vi "Extract message by Rotator.vi"(8 "error in (no error)":errorcluster, 9 "timeout in ms (-1)":i32=-1, 10 "Initialized?":bool, 11 "Queue in":refnum<queue>) -> (0 "error out":errorcluster, 1 "Unread":i32, 2 "Data":variant, 3 "Command out":T1)   [LabVIEW 2024, in "SampleRotator.lvlib"]
doc: "Opens message send by top/master contoller. Reads command and if module was not initialized, it will change any other command than \"Initialize\" into \"Ignore\". \n\nInputs:\nmailbox ref; Initialized?; timeout; error cluster\n\nOutputs:\nCommand; Data; number of unread messages; error cluster"
uses:
  SampleRotator.lvlib
  ctl/Rotator commands.ctl
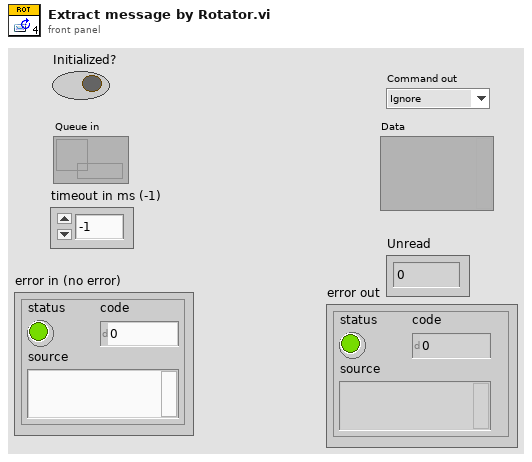
[diagram p1: front panel]
types:
  T1 = typedef "SampleRotator.lvlib/Rotator commands.ctl" = enum16{"Ignore", "Initialize", "Update", "Set parameters", "Stop movement", "Set position", "Disconnect", "End"}
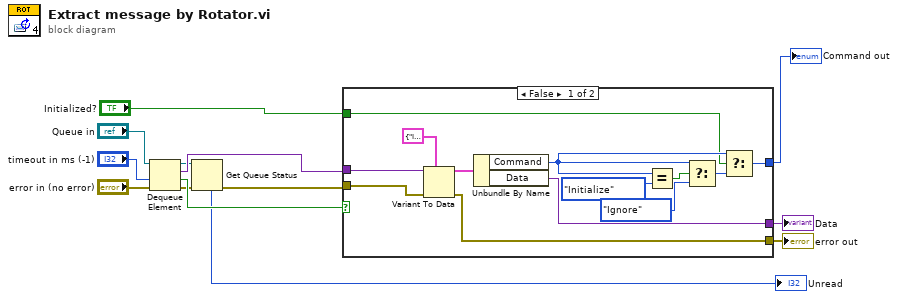
[diagram p0: block diagram]
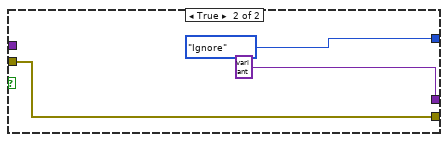
[diagram p2: hidden frame]
diagram:
  n1 = Dequeue Element(queue="Queue in", timeout in ms (-1)="timeout in ms (-1)", error in (no error)="error in (no error)") -> (queue out=w1:refnum<queue>, element=w10:variant, timed out?=w9:bool, error out=w2:errorcluster)
  n2 = Get Queue Status(queue=w1, error in (no error)=w2) -> (error out=w11:errorcluster, # elements in queue=→"Unread":i32)  [unwired: 1 in, 6 out]
  n3 = case shown="False" w9 {
    tunnel: w11 -> [w26 w27]
    tunnel: [w25 w27] -> w3
    tunnel: [w24 variant ("Data")] -> w5
    tunnel: [w23 Rotator_commands."Ignore" ("Command in")] -> w13
    tunnel: w10 -> [w19 _]
    tunnel: "Initialized?" -> [w14 _]
    frame False {
      n4 = Variant To Data(error in=w26, type=cluster{"Command":T1, "Data":variant} {"Command"=enum."Initialize", "Data"=variant} ("MSG to rotator"), Variant=w19) -> (data=w21:cluster{"Command":T1, "Data":variant}, error out=w25:errorcluster)
      n5 = Unbundle By Name(w21) -> ("Command"=w22:T1, "Data"=w24:variant)
      n6 = Equal?(x=w22, y=Rotator_commands."Initialize" ("Command in")) -> (x = y?=w16:bool)
      n7 = Select(t=w22, s=w16, f=Rotator_commands."Ignore" ("Command in")) -> (s? t:f=w15:T1)
      n8 = Select(t=w22, s=w14, f=w15) -> (s? t:f=w23:T1)
    }
    frame True {
    }
  }
  "Command out" <- w13
  "Data" <- w5
  "error out" <- w3
